vi "brc_daq_get_module_info.vi"(0 "index":i32) -> (14 "pModuleInfo_cluster":T1, 19 "error out":errorcluster)   [LabVIEW 2019, in "BRC-DAQ x86.lvlib"]
uses:
  BRC-DAQ x86.lvlib
  brc_daq_pModuleInfo.ctl
  DLL/brc_daq_sdk.dll
panel:
  out "pModuleInfo_string":string
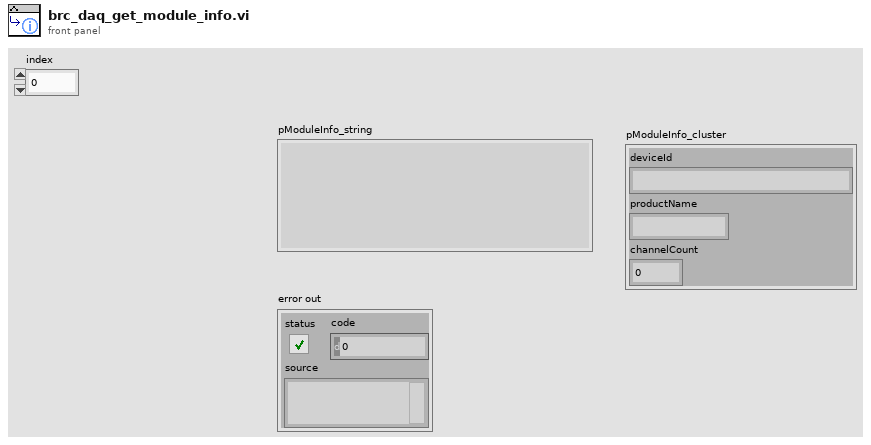
[diagram p1: front panel]
types:
  T1 = typedef "BRC-DAQ x86.lvlib/brc_daq_pModuleInfo.ctl" = cluster{"deviceId":string, "productName":string, "channelCount":i32}
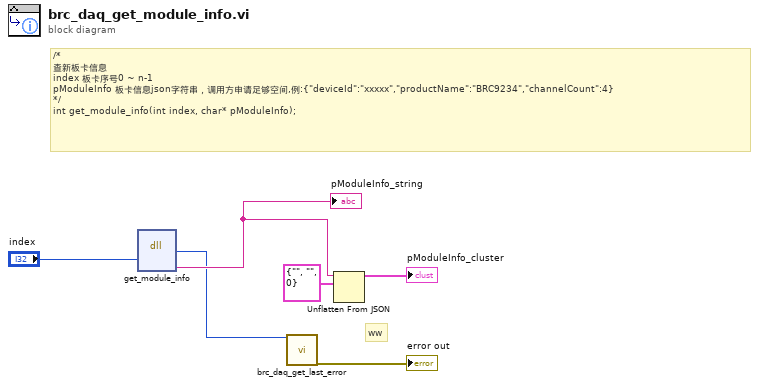
[diagram p0: block diagram]
diagram:
  # "ww"
  # "/*\n查新板卡信息\nindex 板卡序号0 ~ n-1\npModuleInfo 板卡信息json字符串，调用方申请足够空间,例:{\"deviceId\":\"xxxxx\",\"productName\":\"BRC9234\",\"channelCount\":4}\n*/\nint get_module_info(int index, char* pModuleInfo);"
  n1 = dll-call lib="E:/01 BRC project/04BRC-daq/04 Drive/BRC-DAQ/DAQ-x64/DLL/brc_daq_sdk.dll" fn="get_module_info"("index"="index") -> ("return type"=w1:i32, "pModuleInfo"=w2:string)  [unwired: 5 in, 2 out]
  "pModuleInfo_string" <- w2
  n2 = call "brc_daq_get_last_error.vi"("return_value"=w1) -> ("error out"=→"error out":errorcluster)  [unwired: 18 in]
  n3 = Unflatten From JSON(JSON string=w2, type and defaults=T1 {"deviceId"="", "productName"="", "channelCount"=0}) -> (value=→"pModuleInfo_cluster":T1)  [unwired: 5 in, 1 out]
